vi "Estimate Posture from Velocity.vi"(9 "dt (s)":dbl=1.0 format="%0.2f", 10 "initial posture":dbl[](array[numeric])=[0.0, 0.0, 0.0], 11 "estimated steering frame velocity":dbl[](array[numeric])=[0.0, 0.0, 0.0]) -> (0 "y out":dbl, 3 "estimated steering frame posture":dbl[](array[numeric]))   [LabVIEW 2011]
doc: "This VI estimates the posture of a robot by integrating the measured velocity.\n\nThe velocity is a three element array consisting of lateral, forward, and angular velocities relative to the robot's frame of reference.\n\nThe posture is a three element array consiting of the X, Y, and angular position relative to a fixed global frame of reference."
uses:
  <vilib>/Analysis/coordinate.llb/2D Cartesian Coordinate Rotation (Scalar).vi
  <vilib>/ptbypt/NI_PtbyPt.lvlib
  <vilib>/Analysis/NI_AALPro.lvlib
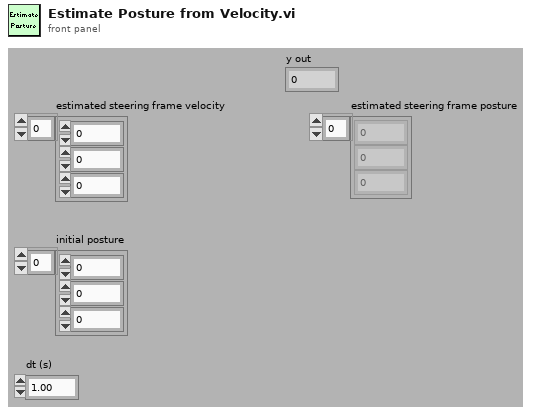
[diagram p1: front panel]
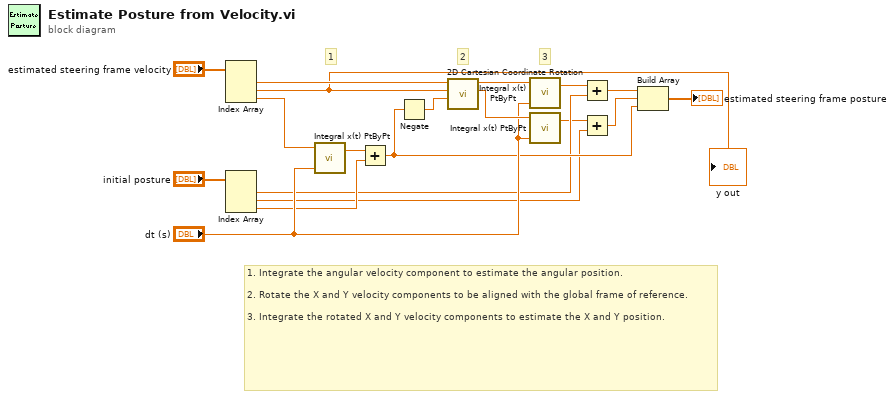
[diagram p0: block diagram]
diagram:
  # "3"
  # "2"
  # "1. Integrate the angular velocity component to estimate the angular position.\n\n2. Rotate the X and Y velocity components to be aligned with the global frame of reference.\n\n3. Integrate the rotated X and Y velocity components to estimate the X and Y position."
  # "1"
  n1 = Index Array(array="estimated steering frame velocity") -> (element #1=w15:dbl, element #2=w1:dbl, element #3=w18:dbl)  [unwired: 3 in]
  "y out" <- w1
  n2 = Index Array(array="initial posture") -> (element #1=w7:dbl, element #2=w4:dbl, element #3=w10:dbl)  [unwired: 3 in]
  n3 = call <vilib>:"Integral x(t) PtByPt.vi"("dt"="dt (s)", "x"=w18) -> ("integral x(t)"=w9:dbl)  [unwired: 2 in, 1 out]
  n4 = Add(x=w9, y=w10) -> (x+y=w8:dbl)
  n5 = Negate(x=w8) -> (-x=w16:dbl)
  n6 = call-poly <vilib>:"2D Cartesian Coordinate Rotation.vi"("theta"=w16, "y"=w1, "x"=w15) -> ("y out"=w13:dbl, "x out"=w14:dbl)  [unwired: 6 in, 1 out]
  n7 = call <vilib>:"Integral x(t) PtByPt.vi"("dt"="dt (s)", "x"=w14) -> ("integral x(t)"=w6:dbl)  [unwired: 2 in, 1 out]
  n8 = call <vilib>:"Integral x(t) PtByPt.vi"("dt"="dt (s)", "x"=w13) -> ("integral x(t)"=w3:dbl)  [unwired: 2 in, 1 out]
  n9 = Add(x=w6, y=w7) -> (x+y=w5:dbl)
  n10 = Add(x=w3, y=w4) -> (x+y=w2:dbl)
  n11 = Build Array(w5, w2, w8) -> (→"estimated steering frame posture":dbl[])
